vi "setState0.vi"(8 "error in (no error)":errorcluster, 10 "State 0 in DOF":dbl[](array[numeric]), 11 "ZTAAC in":refnum<class "ZTAAC.lvclass">) -> (0 "error out":errorcluster, 3 "ZTAAC out":refnum<class "ZTAAC.lvclass">)   [LabVIEW 2016, in "ZTAAC.lvclass"]
doc: "Set the state 0 in degree of freedom (DOF)."
uses:
  ZTAAC.lvclass
  ZTAAC.lvclass/ZTAAC.ctl
  OptCtrl/OptCtrl.lvclass
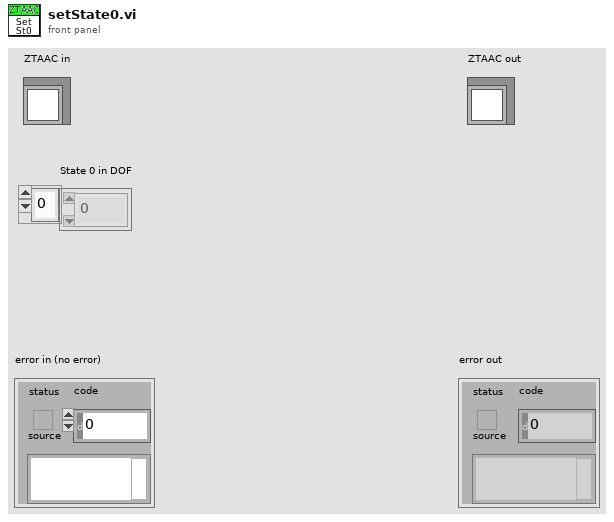
[diagram p1: front panel]
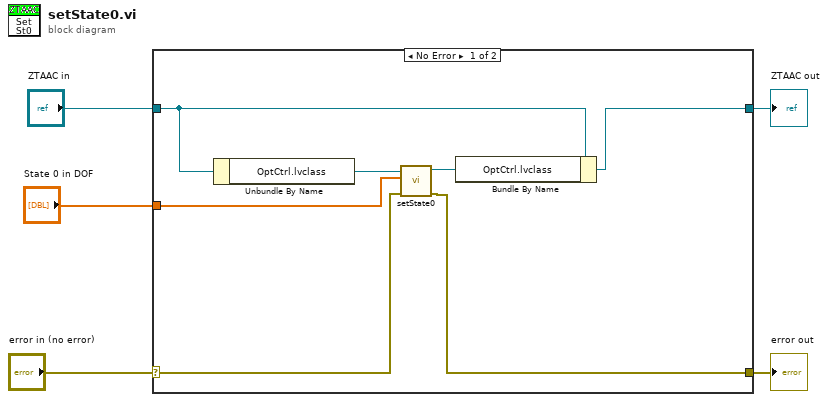
[diagram p0: block diagram]
diagram:
  n1 = case shown="No Error" "error in (no error)" {
    selector: "error in (no error)" -> [w7 w14]
    tunnel: [w6 w14] -> w4
    tunnel: [w8 w13] -> w2
    tunnel: "ZTAAC in" -> [w10 w13]
    tunnel: "State 0 in DOF" -> [w11 _]
    frame No Error {
      n2 = Unbundle By Name(w10) -> ("OptCtrl.lvclass"=w12:refnum<class "OptCtrl.lvclass">)
      n3 = call "setState0.vi"("error in (no error)"=w7, "State 0 in DOF"=w11, "OptCtrl in"=w12) -> ("error out"=w6:errorcluster, "OptCtrl out"=w9:refnum<class "OptCtrl.lvclass">)  [unwired: 7 in]
      n4 = Bundle By Name(cluster=w10, "OptCtrl.lvclass"=w9) -> (w8:refnum<class "ZTAAC.lvclass">)
    }
    frame Error {
    }
  }
  "error out" <- w4
  "ZTAAC out" <- w2
